vi "Text Viewer.vi"(8 "error in":errorcluster, 11 "Path":path) -> (0 "error out":errorcluster, 3 "text out":string)   [LabVIEW 2020]
panel:
  in  "btn save":bool
  in  "btn ok":bool
  in  "Content":string
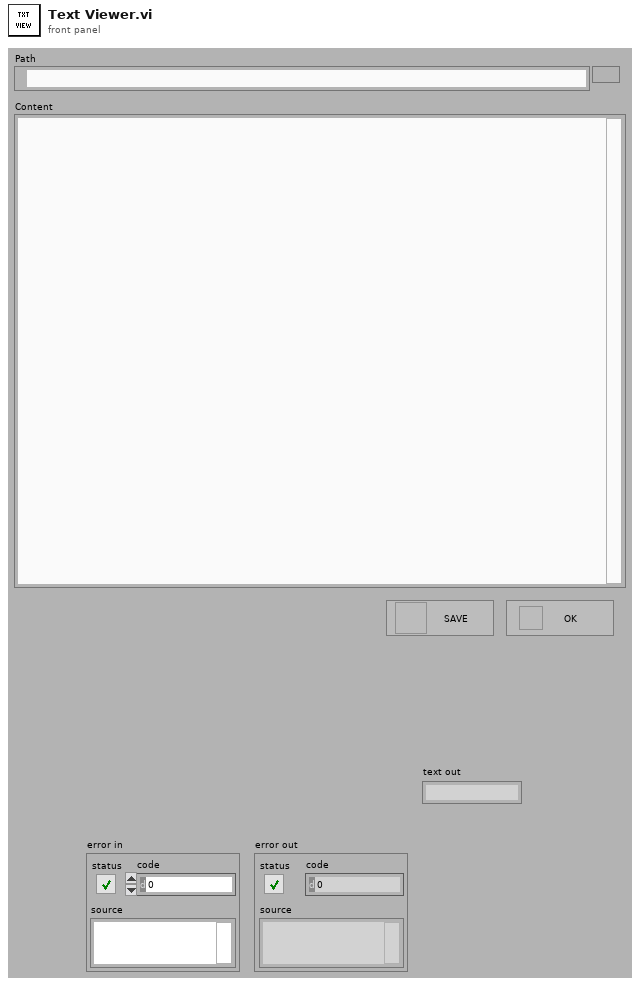
[diagram p1: front panel]
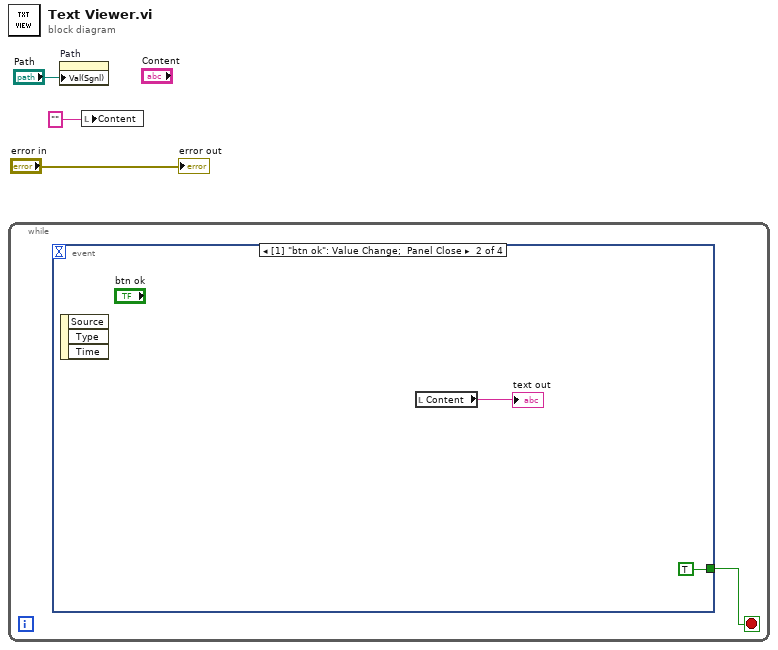
[diagram p0: block diagram]
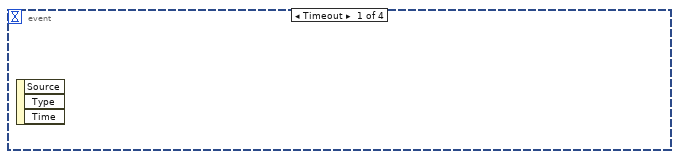
[diagram p2: hidden frame]
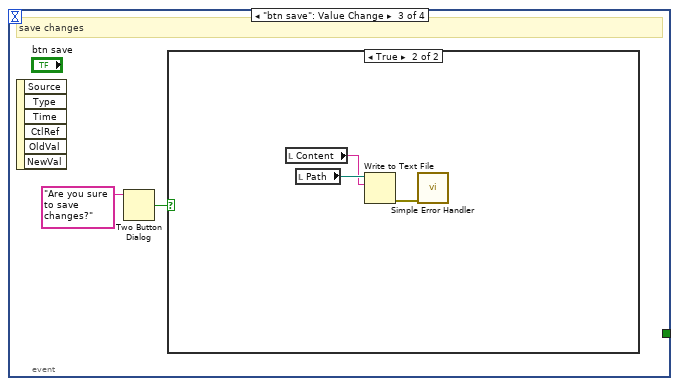
[diagram p3: hidden frame]
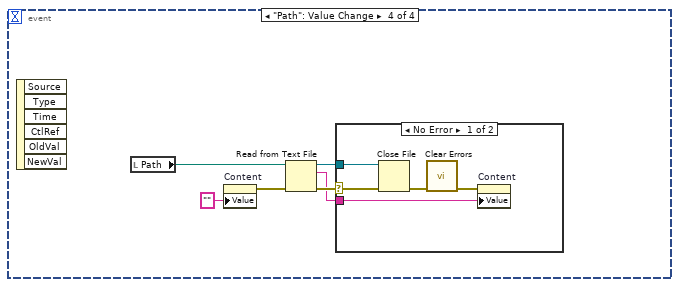
[diagram p5: hidden frame]
diagram:
  n1 = while {
    stop <- w4 stop-if-true
    n2 = event shown="[1] \"btn ok\": Value Change;  Panel Close" {
      selector: _ -> [_ _ _ _]
      dyn-events: _ -> [_ _ _ _]
      timeout: _ -> [_ _ _ _]
      tunnel: [_ TRUE _ _] -> w4
      event Timeout {
        n3 = event-data() -> ()  [unwired: 1 in, 3 out]
      }
      event "btn ok": Value Change; Panel Close {
        n4 = event-data() -> ()  [unwired: 1 in, 3 out]
        n5 = local read "Content"() -> (→"text out":string)
      }
      event "btn save": Value Change {
        # "save changes"
        n6 = event-data() -> ()  [unwired: 1 in, 6 out]
        n7 = Two Button Dialog(message="Are you sure to save changes?") -> (T button?=w8:bool)  [unwired: 2 in]
        n8 = case shown="True" w8 {
          frame False {
          }
          frame True {
            n9 = local read "Content"() -> (w10:string)
            n10 = local read "Path"() -> (w11:path)
            n11 = Write to Text File(file (use dialog)=w11, text=w10) -> (error out=w9:errorcluster)  [unwired: 2 in, 2 out]
            n12 = call <vilib>:"Simple Error Handler.vi"("error in (no error)"=w9) -> ()  [unwired: 4 in, 5 out]
          }
        }
      }
      event "Path": Value Change {
        n13 = event-data() -> ()  [unwired: 1 in, 6 out]
        n14 = local read "Path"() -> (w17:path)
        n15 = property on="Content" class="Str"("Value"="" ("Content")) -> (error out=w16:errorcluster)  [unwired: 2 in, 1 out]
        n16 = Read from Text File(file (use dialog)=w17, error in=w16) -> (refnum out=w13:refnum<file>, text=w12:string, error out=w14:errorcluster)  [unwired: 2 in, 1 out]
        n17 = case shown="No Error" w14 {
          selector: w14 -> [w22 _]
          tunnel: w13 -> [w21 _]
          tunnel: w12 -> [w18 _]
          frame No Error {
            n18 = Close File(refnum=w21, error in=w22) -> (error out=w20:errorcluster)  [unwired: 1 out]
            n19 = call <vilib>:"Clear Errors.vi"("error in (no error)"=w20) -> ("error out"=w19:errorcluster)  [unwired: 5 in, 1 out]
            n20 = property on="Content" class="Str"(error in=w19, "Value"=w18) -> ()  [unwired: 1 in, 2 out]
          }
          frame Error {
          }
        }
      }
    }
  }
  n21 = property on="Path" class="Path"("Val(Sgnl)"="Path") -> ()  [unwired: 2 in, 2 out]
  n22 = local write "Content"("" ("Content")) -> ()
  "error out" <- "error in"
